vi "fpga_FIFO control (M Class_60Hz).vi"(0 "Time stamp":fxp<+,64,32> format="%.42g", 1 "reset":bool, 2 "filter delay constant":T1=enum."60Hz:10 reporting rate", 5 "Frequency":fxp<+,32,8>, 7 "#ch":fxp<+,5,5>, 9 "PMU VI input valid":bool, 11 "PMU VI output valid":bool) -> (4 "Time Stamp out":fxp<+,64,32> format="%.42g", 14 "data valid?":bool, 15 "Frequency output":fxp<+,32,8> format="%.27g")   [LabVIEW 2013, in "NI_EP_PMU_FPGA.lvlib"]
uses:
  <vilib>/addons/Electrical Power/PMU/NI_EP_PMU_FPGA.lvlib
  <vilib>/addons/Electrical Power/PMU/FPGA/subVIs/fpga_Reporting Rate Configuration.ctl
  <vilib>/rvi/DataTransferAndStorage/Container/Common/niFpgaContainerGetUniqueNameForEmu.vi
  <vilib>/rvi/DataTransferAndStorage/Container/Common/niFpgaContainerSetEmuInfo.vi
  <vilib>/rvi/eio/common/nirviEmuReportErrorAndStop.vi
  <vilib>/rvi/FIFO/Fifo_Resource/nirvififoEmulationWriteFpgaImpl.vi
  <vilib>/rvi/FIFO/Fifo_Resource/nirvififoEmulationReadFpgaImpl.vi
  <vilib>/rvi/LocalResourceManager/LocalResourceManager.xnode
  <vilib>/rvi/DataTransferAndStorage/Container/XNode/niFpgaContainer.xnode
  <vilib>/rvi/FIFO/Fifo_Resource/nirvififoEmulationWrite.vi
  <vilib>/rvi/FXPMathLib/FxpSub/XNode/nifxpmath_Sub.xnode
  <vilib>/rvi/FXPMathLib/basic elements/FxpDiscreteDelay/XNode/nifxpmath_DiscreteDelay.xnode
  <vilib>/rvi/FIFO/Fifo_Resource/nirvififoEmulationRead.vi
  <vilib>/addons/Electrical Power/PQ/Resampling/NI_EP_Resample_FPGA.lvlib
  <vilib>/rvi/FXPMathLib/sim/FxpSim.dll
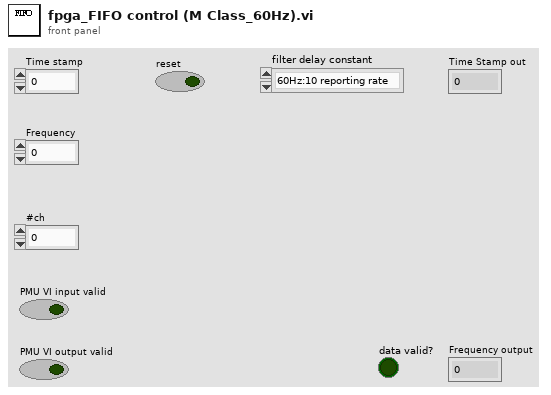
[diagram p1: front panel]
types:
  T1 = typedef "NI_EP_PMU_FPGA.lvlib/fpga_Reporting Rate Configuration.ctl" = enum16{"50Hz:50 reporting rate", "50Hz:25 reporting rate", "50Hz:10 reporting rate", "60Hz:60 reporting rate", "60Hz:30 reporting rate", "60Hz:20 reporting rate", "60Hz:15 reporting rate", "60Hz:12 reporting rate", "60Hz:10 reporting rate"}
  T2 = cluster{"frequency":fxp<+,32,8>, "timestamp":fxp<+,64,32>}
  T3 = cluster{"frequency":fxp<+,32,8>, "timestamp":fxp<+,64,32>}[]
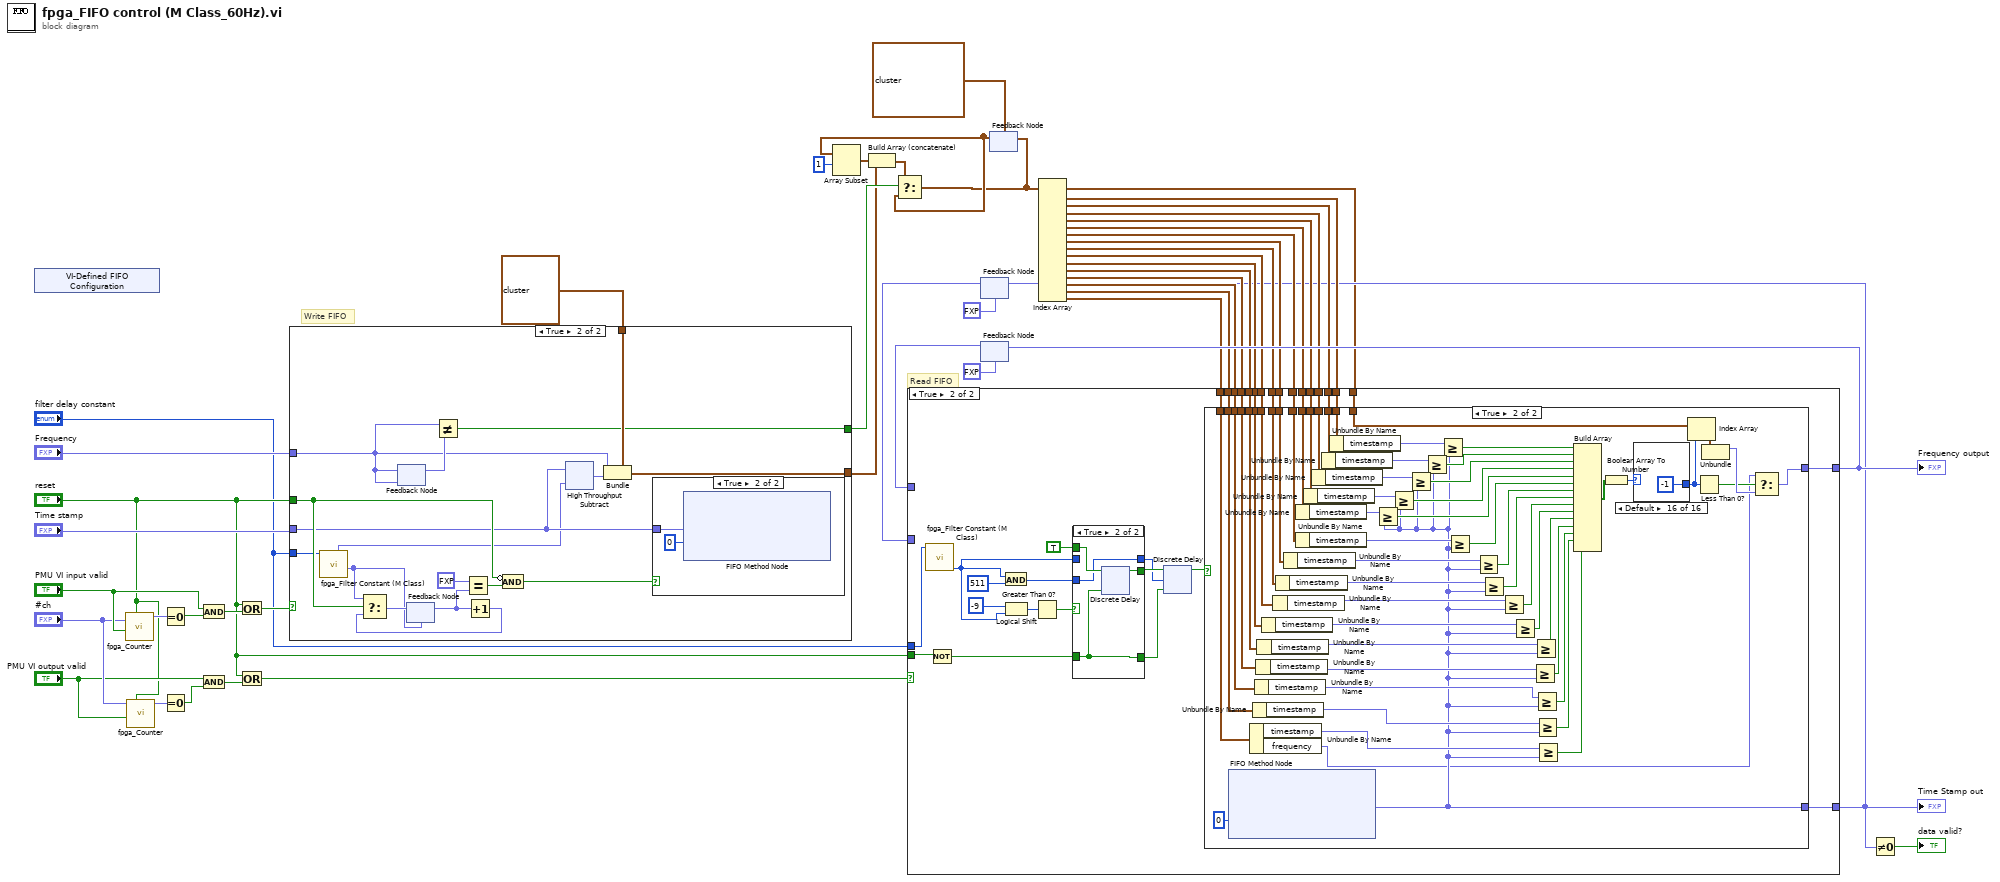
[diagram p0: block diagram]
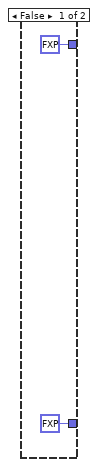
[diagram p4: hidden frame]
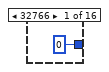
[diagram p5: hidden frame]
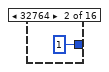
[diagram p6: hidden frame]
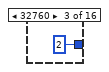
[diagram p7: hidden frame]
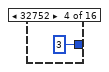
[diagram p8: hidden frame]
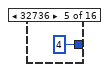
[diagram p9: hidden frame]
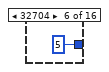
[diagram p10: hidden frame]
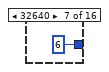
[diagram p11: hidden frame]
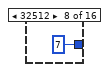
[diagram p12: hidden frame]
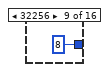
[diagram p13: hidden frame]
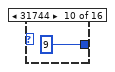
[diagram p14: hidden frame]
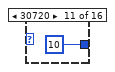
[diagram p15: hidden frame]
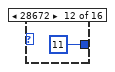
[diagram p16: hidden frame]
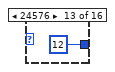
[diagram p17: hidden frame]
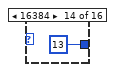
[diagram p18: hidden frame]
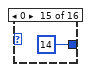
[diagram p19: hidden frame]
diagram:
  # "Read FIFO"
  # "Write FIFO"
  n1 = xnode "VI-Defined FIFO Configuration"() -> ()  [unwired: 1 out]
  n2 = call <vilib>:"fpga_Counter.vi"("reset"="reset", "Input Valid?"="PMU VI input valid", "upper limit"="#ch") -> ("count"=w34:fxp<+,5,5>)  [unwired: 7 in, 1 out]
  n3 = call <vilib>:"fpga_Counter.vi"("reset"="reset", "Input Valid?"="PMU VI output valid", "upper limit"="#ch") -> ("count"=w33:fxp<+,5,5>)  [unwired: 7 in, 1 out]
  n4 = Equal To 0?(x=w34) -> (x = 0?=w45:bool)
  n5 = Equal To 0?(x=w33) -> (x = 0?=w41:bool)
  n6 = And(x="PMU VI input valid", y=w45) -> (x .and. y?=w38:bool)
  n7 = And(x="PMU VI output valid", y=w41) -> (x .and. y?=w44:bool)
  n8 = Or(x="reset", y=w38) -> (x .or. y?=w37:bool)
  n9 = Or(x="reset", y=w44) -> (x .or. y?=w43:bool)
  n10 = case shown="True" w37 {
    tunnel: "Time stamp" -> [_ w50]
    tunnel: "reset" -> [_ w58]
    tunnel: "Frequency" -> [_ w49]
    tunnel: [_ w51] -> w25
    tunnel: [_ w53] -> w24
    tunnel: T2 {"frequency"=0.0, "timestamp"=0.0} -> [_ w52]
    tunnel: "filter delay constant" -> [_ w48]
    frame False {
    }
    frame True {
      n11 = call <vilib>:"fpga_Filter Constant (M Class).vi"("filter delay constant"=w48) -> ("Start"=w57:fxp<+/-,4,4>, "reference delay"=w47:fxp<+,22,0>)  [unwired: 6 in, 3 out]
      n12 = feedback #1(w49) -> (w55:fxp<+,32,8>)
      n13 = feedback-in #1(w49) -> ()
      n14 = feedback #2(w57) -> (w61:fxp<+/-,4,4>)
      n15 = Not Equal?(x=w49, y=w55) -> (x != y?=w51:bool)
      n16 = Equal?(x=fxp<+/-,4,4> 7.0, y=w61) -> (x = y?=w59:bool)
      n17 = Increment(x=w61) -> (x+1=w62:fxp<+,3,3>)
      n18 = Select(t=w57, s=w58, f=w62) -> (s? t:f=w63:fxp<+/-,4,4>)
      n19 = feedback-in #2(w63) -> ()
      n20 = Compound Arithmetic op=AND(invert w58, w59) -> (w56:bool)
      n21 = xnode "High Throughput Subtract"("x"=w50, "y"=w47) -> ("x-y"=w54:fxp<+,64,32>)
      n22 = Bundle(cluster=w52, "frequency"=w49, "timestamp"=w54) -> (w53:T2)
      n23 = case shown="True" w56 {
        tunnel: w50 -> [_ w64]
        frame False {
        }
        frame True {
          n24 = xnode ("FIFO Method Node")("Element"=w64, "Timeout"=0) -> ()  [unwired: 1 in, 2 out]
        }
      }
    }
  }
  n25 = feedback #3(fxp<+,64,32> 0.0 ("Element")) -> (w42:fxp<+,64,32>)
  n26 = feedback #4(fxp<+,32,8> 0.0 ("Element")) -> (w39:fxp<+,32,8>)
  n27 = feedback #5(T3 [{"frequency"=0.0, "timestamp"=0.0}, {"frequency"=0.0, "timestamp"=0.0}, {"frequency"=0.0, "timestamp"=0.0}, {"frequency"=0.0, "timestamp"=0.0}, {"frequency"=0.0, "timestamp"=0.0}, {"frequency"=0.0, "timestamp"=0.0}, {"frequency"=0.0, "timestamp"=0.0}, {"frequency"=0.0, "timestamp"=0.0}, {"frequency"=0.0, "timestamp"=0.0}, {"frequency"=0.0, "timestamp"=0.0}, {"frequency"=0.0, "timestamp"=0.0}, {"frequency"=0.0, "timestamp"=0.0}, {"frequency"=0.0, "timestamp"=0.0}, {"frequency"=0.0, "timestamp"=0.0}, {"frequency"=0.0, "timestamp"=0.0}]) -> (w13:T3)
  n28 = Array Subset(array=w13, index=1) -> (w26:T3)  [unwired: 1 in]
  n29 = Build Array (concatenate)(w26, w24) -> (w16:T3)
  n30 = Select(t=w16, s=w25, f=w13) -> (s? t:f=w1:T3)
  n31 = feedback-in #5(w1) -> ()
  n32 = Index Array(array=w1) -> (element #1=w23:T2, element #2=w22:T2, element #3=w21:T2, element #4=w20:T2, element #5=w19:T2, element #6=w15:T2, element #7=w14:T2, element #8=w12:T2, element #9=w11:T2, element #10=w9:T2, element #11=w10:T2, element #12=w8:T2, element #13=w7:T2, element #14=w6:T2, element #15=w5:T2)  [unwired: 15 in]
  n33 = case shown="True" w43 {
    tunnel: "reset" -> [_ w97]
    tunnel: [w67 w99] -> w3
    tunnel: w42 -> [w67 _]
    tunnel: [w66 w98] -> w29
    tunnel: w39 -> [w66 _]
    tunnel: w23 -> [_ w96]
    tunnel: w22 -> [_ w95]
    tunnel: w21 -> [_ w94]
    tunnel: w20 -> [_ w93]
    tunnel: w19 -> [_ w92]
    tunnel: w1 -> [_ w91]
    tunnel: w15 -> [_ w90]
    tunnel: w14 -> [_ w89]
    tunnel: w12 -> [_ w88]
    tunnel: w11 -> [_ w87]
    tunnel: w9 -> [_ w86]
    tunnel: "filter delay constant" -> [_ w85]
    tunnel: w10 -> [_ w84]
    tunnel: w8 -> [_ w83]
    tunnel: w7 -> [_ w82]
    tunnel: w6 -> [_ w81]
    tunnel: w5 -> [_ w80]
    frame False {
    }
    frame True {
      n34 = call <vilib>:"fpga_Filter Constant (M Class).vi"("filter delay constant"=w85) -> ("Total Delay"=w74:u16)  [unwired: 6 in, 4 out]
      n35 = Not(x=w97) -> (.not. x?=w78:bool)
      n36 = And(x=w74, y=u16 511) -> (x .and. y?=w76:u16)
      n37 = Logical Shift(y=i16 -9, x=w74) -> (x << y=w73:u16)
      n38 = Greater Than 0?(x=w73) -> (x > 0?=w72:bool)
      n39 = case shown="True" w72 {
        tunnel: TRUE ("D") -> [w102 w105]
        tunnel: [w102 w106] -> w71
        tunnel: w78 -> [w101 w104]
        tunnel: w76 -> [_ w103]
        tunnel: w74 -> [w100 _]
        tunnel: [w101 w104] -> w70
        tunnel: [w100 w103] -> w69
        frame False {
        }
        frame True {
          n40 = xnode ("Discrete Delay")("D"=w105, "enable"=w104) -> ("Q"=w106:bool)
        }
      }
      n41 = xnode ("Discrete Delay")("D"=w71, "n-1[0..511]"=w69, "enable"=w70) -> ("Q"=w68:bool)
      n42 = case shown="True" w68 {
        tunnel: [fxp<+,64,32> 0.0 ("Element") w115] -> w99
        tunnel: [fxp<+,32,8> 0.0 ("frequency") w138] -> w98
        tunnel: w96 -> [_ w159]
        tunnel: w95 -> [_ w160]
        tunnel: w94 -> [_ w161]
        tunnel: w93 -> [_ w162]
        tunnel: w92 -> [_ w163]
        tunnel: w91 -> [_ w153]
        tunnel: w90 -> [_ w145]
        tunnel: w89 -> [_ w142]
        tunnel: w88 -> [_ w136]
        tunnel: w87 -> [_ w135]
        tunnel: w86 -> [_ w134]
        tunnel: w84 -> [_ w125]
        tunnel: w83 -> [_ w124]
        tunnel: w82 -> [_ w123]
        tunnel: w81 -> [_ w122]
        tunnel: w80 -> [_ w121]
        frame False {
        }
        frame True {
          n43 = xnode ("FIFO Method Node")("Timeout"=0) -> ("Element"=w115:fxp<+,64,32>)  [unwired: 1 in, 2 out]
          n44 = Unbundle By Name(w121) -> ("timestamp"=w116:fxp<+,64,32>, "frequency"=w109:fxp<+,32,8>)
          n45 = Unbundle By Name(w122) -> ("timestamp"=w117:fxp<+,64,32>)
          n46 = Unbundle By Name(w123) -> ("timestamp"=w118:fxp<+,64,32>)
          n47 = Unbundle By Name(w124) -> ("timestamp"=w119:fxp<+,64,32>)
          n48 = Unbundle By Name(w125) -> ("timestamp"=w120:fxp<+,64,32>)
          n49 = Unbundle By Name(w134) -> ("timestamp"=w128:fxp<+,64,32>)
          n50 = Unbundle By Name(w135) -> ("timestamp"=w131:fxp<+,64,32>)
          n51 = Unbundle By Name(w136) -> ("timestamp"=w133:fxp<+,64,32>)
          n52 = Unbundle By Name(w142) -> ("timestamp"=w141:fxp<+,64,32>)
          n53 = Unbundle By Name(w163) -> ("timestamp"=w158:fxp<+,64,32>)
          n54 = Unbundle By Name(w145) -> ("timestamp"=w144:fxp<+,64,32>)
          n55 = Unbundle By Name(w162) -> ("timestamp"=w157:fxp<+,64,32>)
          n56 = Unbundle By Name(w161) -> ("timestamp"=w156:fxp<+,64,32>)
          n57 = Unbundle By Name(w160) -> ("timestamp"=w155:fxp<+,64,32>)
          n58 = Unbundle By Name(w159) -> ("timestamp"=w154:fxp<+,64,32>)
          n59 = Greater Or Equal?(x=w158, y=w115) -> (x >= y?=w148:bool)
          n60 = Greater Or Equal?(x=w157, y=w115) -> (x >= y?=w149:bool)
          n61 = Greater Or Equal?(x=w156, y=w115) -> (x >= y?=w150:bool)
          n62 = Greater Or Equal?(x=w155, y=w115) -> (x >= y?=w151:bool)
          n63 = Greater Or Equal?(x=w154, y=w115) -> (x >= y?=w152:bool)
          n64 = Greater Or Equal?(x=w144, y=w115) -> (x >= y?=w143:bool)
          n65 = Greater Or Equal?(x=w141, y=w115) -> (x >= y?=w140:bool)
          n66 = Greater Or Equal?(x=w133, y=w115) -> (x >= y?=w132:bool)
          n67 = Greater Or Equal?(x=w131, y=w115) -> (x >= y?=w130:bool)
          n68 = Greater Or Equal?(x=w128, y=w115) -> (x >= y?=w129:bool)
          n69 = Greater Or Equal?(x=w119, y=w115) -> (x >= y?=w113:bool)
          n70 = Greater Or Equal?(x=w120, y=w115) -> (x >= y?=w114:bool)
          n71 = Greater Or Equal?(x=w118, y=w115) -> (x >= y?=w112:bool)
          n72 = Greater Or Equal?(x=w117, y=w115) -> (x >= y?=w111:bool)
          n73 = Greater Or Equal?(x=w116, y=w115) -> (x >= y?=w110:bool)
          n74 = Build Array(w152, w151, w150, w149, w148, w143, w140, w132, w130, w129, w114, w113, w112, w111, w110) -> (w147:bool[])
          n75 = Boolean Array To Number(Boolean array=w147) -> (number=w127:u16)
          n76 = case shown="Default" w127 {
            tunnel: [0 ("index") 1 ("index") 2 ("index") 3 ("index") 4 ("index") 5 ("index") 6 ("index") 7 ("index") 8 ("index") 9 ("index") 10 ("index") 11 ("index") 12 ("index") 13 ("index") 14 ("index") -1 ("index")] -> w126
            frame 32766 {
            }
            frame 32764 {
            }
            frame 32760 {
            }
            frame 32752 {
            }
            frame 32736 {
            }
            frame 32704 {
            }
            frame 32640 {
            }
            frame 32512 {
            }
            frame 32256 {
            }
            frame 31744 {
            }
            frame 30720 {
            }
            frame 28672 {
            }
            frame 24576 {
            }
            frame 16384 {
            }
            frame 0 {
            }
            frame Default {
            }
          }
          n77 = Index Array(array=w153, index=w126) -> (element=w146:T2)
          n78 = Less Than 0?(x=w126) -> (x < 0?=w137:bool)
          n79 = Unbundle(w146) -> ("frequency"=w139:fxp<+,32,8>)  [unwired: 1 out]
          n80 = Select(t=w109, s=w137, f=w139) -> (s? t:f=w138:fxp<+,32,8>)
        }
      }
    }
  }
  "Time Stamp out" <- w3
  "Frequency output" <- w29
  n81 = feedback-in #3(w3) -> ()
  n82 = feedback-in #4(w29) -> ()
  n83 = Not Equal To 0?(x=w3) -> (x != 0?=→"data valid?":bool)
